vi "SMC_setup.vi"(0 "VISA Resource Name":refnum<visa-resource-name>, 5 "Mixer file (*.mxr)":path, 7 "Format":string(combo)="MLINear", 9 "Measurement":string(combo)="SC21", 11 "error in (no error)":errorcluster, 12 "Channel":i32=1) -> (4 "dup VISA session":refnum<visa-resource-name>, 8 "Filename":string="Mixer", 15 "error out":errorcluster)   [LabVIEW 2018]
uses:
  Instance           2 17Saved   SMC_setup .vi
  Instance           1 17Saved   SMC_setup .vi
  PNA-X.lvlib
panel:
  # "The Mixer file must be stored locally on the PNA"
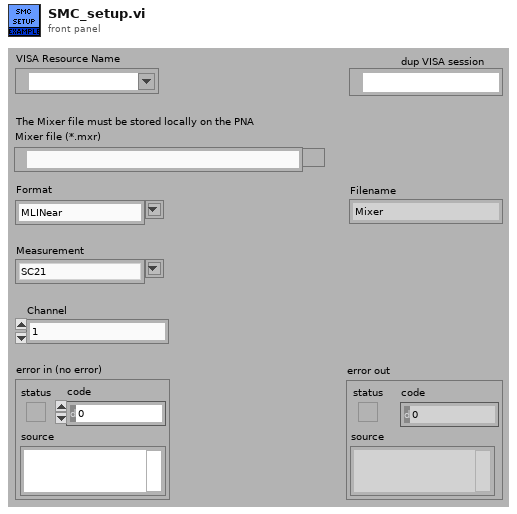
[diagram p1: front panel]
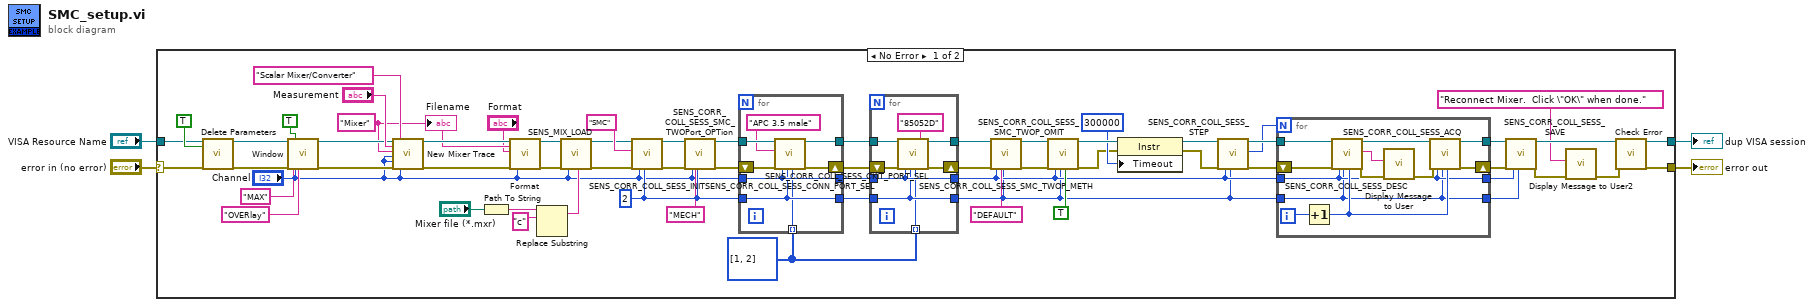
[diagram p0: block diagram]
diagram:
  n1 = case shown="No Error" "error in (no error)" {
    selector: "error in (no error)" -> [w8 w96]
    tunnel: [w48 w97] -> w4
    tunnel: [w47 w96] -> w3
    tunnel: "VISA Resource Name" -> [w46 w97]
    frame No Error {
      w50 = i32[] [1, 2]
      w35 = 2 ("Session")
      w10 = "Mixer" ("Measurement Name")
      n2 = call "Delete Parameters .vi"("VISA IN"=w46, "Delete All?"=TRUE, "error in"=w8) -> ("VISA Out"=w44:refnum<visa-resource-name>, "error out"=w43:errorcluster)  [unwired: 15 in]
      n3 = call "Window.vi"("VISA IN"=w44, "error in"=w43, "Window\nCreate(ON)/Delete(OFF)"=TRUE ("Window\nCreate(ON)/Delete(OFF)"), "Window"="Channel", "Window Size"="MAX", "Window Arrangement"="OVERlay") -> ("VISA Out"=w42:refnum<visa-resource-name>, "error out"=w41:errorcluster)  [unwired: 12 in]
      n4 = call "New Mixer Trace.vi"("VISA IN"=w42, "Meas Param"="Measurement", "FileName"=w10, "Window"="Channel", "Trace"="Channel", "error in (no error)"=w41, "Meas Type"="Scalar Mixer/Converter" ("Measurement Type"), "Channel"="Channel") -> ("VISA Out"=w13:refnum<visa-resource-name>, "error out"=w15:errorcluster)  [unwired: 10 in]
      n5 = Path To String(path="Mixer file (*.mxr)") -> (string=w17:string)
      n6 = call "Format.vi"("VISA IN"=w13, "Measurement Name"=w10, "Format"="Format", "error in"=w15, "Channel"="Channel") -> ("VISA Out"=w12:refnum<visa-resource-name>, "error out"=w14:errorcluster)  [unwired: 13 in]
      n7 = Replace Substring(4:"c" ("substring (\"\")"), 5:w17) -> (1:w16:string)  [unwired: 2 in, 1 out]
      n8 = call "SENS_MIX_LOAD.vi"("VISA IN"=w12, "error in"=w14, "Channel"="Channel", "FileName"=w16) -> ("VISA Out"=w29:refnum<visa-resource-name>, "error out"=w28:errorcluster)  [unwired: 14 in]
      n9 = call "SENS_CORR_COLL_SESS_INIT.vi"("VISA IN"=w29, "ClaType"="SMC", "error in"=w28, "Channel"="Channel", "Session"=w35) -> ("VISA Out"=w27:refnum<visa-resource-name>, "error out"=w26:errorcluster)  [unwired: 13 in]
      n10 = call "SENS_CORR_COLL_SESS_SMC_TWOPort_OPTion.vi"("VISA IN"=w27, "error in"=w26, "Channel"="Channel", "Session"=w35, "CalType"="MECH") -> ("VISA Out"=w54:refnum<visa-resource-name>, "error out"=w53:errorcluster)  [unwired: 13 in]
      n11 = for {
        tunnel: w54 -> [w75]
        tunnel: [w74] -> w25
        shift-right: [w72] -> w24
        shift-left: w53 -> [w73]
        tunnel: "Channel" -> [w71]
        tunnel: [w71] -> w52
        tunnel: w35 -> [w70]
        tunnel: [w70] -> w51
        tunnel: w50 -> [w68] mode=indexing
        n12 = call "SENS_CORR_COLL_SESS_CONN_PORT_SEL.vi"("VISA IN"=w75, "ConnType"="APC 3.5 male", "error in"=w73, "Channel"=w71, "Session"=w70, "Port"=w68) -> ("VISA Out"=w74:refnum<visa-resource-name>, "error out"=w72:errorcluster)  [unwired: 12 in]
      }
      n13 = for {
        shift-right: [w92] -> w22
        shift-left: w24 -> [w95]
        tunnel: w52 -> [w91]
        tunnel: w51 -> [w90]
        tunnel: w50 -> [w88] mode=indexing
        tunnel: [w94] -> w23
        tunnel: [w91] -> w37
        tunnel: [w90] -> w36
        tunnel: w25 -> [w89]
        n14 = call "SENS_CORR_COLL_SESS_CKIT_PORT_SEL.vi"("VISA IN"=w89, "error in"=w95, "Channel"=w91, "Session"=w90, "Port"=w88, "CalKit"="85052D") -> ("VISA Out"=w94:refnum<visa-resource-name>, "error out"=w92:errorcluster)  [unwired: 12 in]
      }
      n15 = call "SENS_CORR_COLL_SESS_SMC_TWOP_METH.vi"("VISA IN"=w23, "error in"=w22, "Channel"=w37, "Session"=w36, "Method"="DEFAULT") -> ("VISA Out"=w21:refnum<visa-resource-name>, "error out"=w20:errorcluster)  [unwired: 13 in]
      n16 = call "SENS_CORR_COLL_SESS_SMC_TWOP_OMIT.vi"("VISA IN"=w21, "error in"=w20, "Channel"=w37, "Session"=w36, "OmitIsol?"=TRUE) -> ("VISA Out"=w34:refnum<visa-resource-name>, "error out"=w31:errorcluster)  [unwired: 13 in]
      n17 = property class="Instr"(reference=w34, error in=w31, "Timeout"=u32 300000 ("General Settings:Timeout Value")) -> (reference out=w33:refnum<visa-resource-name>, error out=w30:errorcluster)
      n18 = call "SENS_CORR_COLL_SESS_STEP.vi"("VISA IN"=w33, "error in"=w30, "Channel"=w37, "Session"=w36) -> ("VISA Out"=w61:refnum<visa-resource-name>, "Step"=w59:i32, "error out"=w60:errorcluster)  [unwired: 13 in]
      n19 = for {
        N: w59 -> [_]
        tunnel: w61 -> [w86]
        shift-right: [w79] -> w57
        shift-left: w60 -> [w85]
        tunnel: [w80] -> w58
        tunnel: w37 -> [w77]
        tunnel: w36 -> [w76]
        tunnel: [w77] -> w56
        tunnel: [w76] -> w55
        i -> [w87]
        n20 = Increment(x=w87) -> (x+1=w78:i32)
        n21 = call "SENS_CORR_COLL_SESS_DESC.vi"("VISA IN"=w86, "error in"=w85, "Channel"=w77, "Session"=w76, "StepNum"=w78) -> ("VISA Out"=w82:refnum<visa-resource-name>, "read buffer"=w84:string, "error out"=w83:errorcluster)  [unwired: 12 in]
        n22 = call "Display Message to User"("error in (no error)"=w83, "Message"=w84) -> ("error out"=w81:errorcluster)  [unwired: 8 in, 1 out]
        n23 = call "SENS_CORR_COLL_SESS_ACQ.vi"("VISA IN"=w82, "error in"=w81, "Channel"=w77, "Session"=w76, "AcqCnt"=w78) -> ("VISA Out"=w80:refnum<visa-resource-name>, "error out"=w79:errorcluster)  [unwired: 13 in]
      }
      n24 = call "SENS_CORR_COLL_SESS_SAVE.vi"("VISA IN"=w58, "error in"=w57, "Channel"=w56, "Session"=w55) -> ("VISA Out"=w49:refnum<visa-resource-name>, "error out"=w7:errorcluster)  [unwired: 14 in]
      n25 = call "Display Message to User2"("error in (no error)"=w7, "Message"="Reconnect Mixer.  Click \"OK\" when done.") -> ("error out"=w6:errorcluster)  [unwired: 8 in, 1 out]
      n26 = call "Check Error.vi"("VISA Resource Name"=w49, "error in (no error)"=w6) -> ("dup VISA session"=w48:refnum<visa-resource-name>, "error out"=w47:errorcluster)  [unwired: 16 in]
      "Filename" <- w10
    }
    frame Error {
    }
  }
  "error out" <- w3
  "dup VISA session" <- w4
